vi "Create.vi"(10 "Groups":refnum<class "Group DBL.lvclass">[](array[class])) -> (3 "GroupsValue out":refnum<class "GroupArrayValue.lvclass">)   [LabVIEW 2020, in "Vecto.lvlib" / "GroupArrayValue.lvclass"]
uses:
  GroupArrayValue.lvclass
  Group DBL/Group DBL.lvclass
  GroupArrayValue.lvclass/GroupArrayValue.ctl
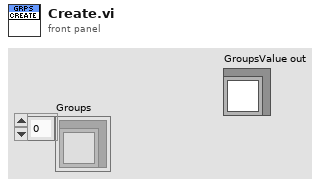
[diagram p1: front panel]
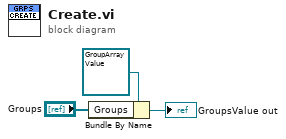
[diagram p0: block diagram]
diagram:
  n1 = Bundle By Name(cluster=refnum<class "GroupArrayValue.lvclass"> refnum ("GroupsValue out"), "Groups"="Groups") -> (→"GroupsValue out":refnum<class "GroupArrayValue.lvclass">)
